vi "Send Message to Azure Queue.vi"() -> ()   [LabVIEW 2015]
doc: "Demonstrates how to send a message to an existing Azure queue."
uses:
  Core/Azure Credentials.ctl
  Core/NI_Azure_Core.lvlib
  Core/Session/Session.lvclass
  Queue/NI_Azure_Queue.lvlib
panel:
  in  "Access Key":string
  in  "Storage Account Name":string
  in  "Queue Name":string
  in  "Message Body":string
  # "Overview: Demonstrates how to send a message to an existing Azure queue.\nRequirements: NI Cloud Toolkit for Azure and a registered Microsoft Azure account\nInstructions:\n1. Specify the Storage Account Name and Access Key for your Azure account. You can create an account at http://azure.microsoft.com.\n2. Specify a Queue Name for the queue to which you want to send a message. You can run the Create New Azure Queue.vi example to create a new queue.\n3. Specify a Message Body to send to the queue.\n4. Run the VI. Verify in the Microsoft Azure Portal that the specified queue has an available message."
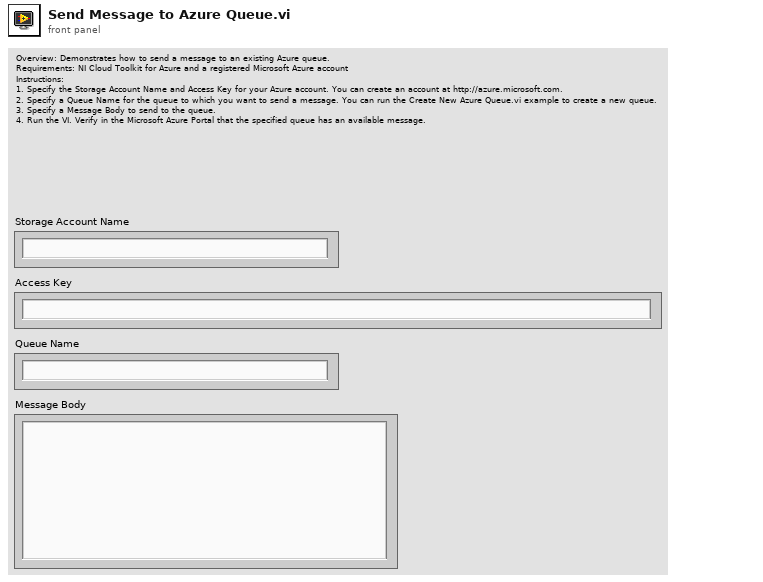
[diagram p1: front panel]
types:
  T1 = typedef "NI_Azure_Core.lvlib/Azure Credentials.ctl" = cluster{"Storage Account Name":string, "Access Key":string}
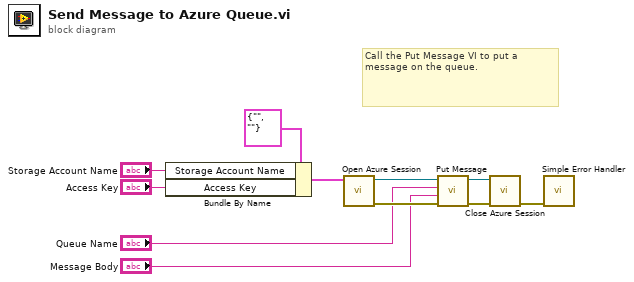
[diagram p0: block diagram]
diagram:
  # "Call the Put Message VI to put a message on the queue."
  n1 = Bundle By Name(cluster=T1 {"Storage Account Name"="", "Access Key"=""} ("Credentials"), "Storage Account Name"="Storage Account Name", "Access Key"="Access Key") -> (w8:T1)
  n2 = call "Open Azure Session.vi"("Credentials"=w8) -> ("error out"=w5:errorcluster, "Azure Session"=w6:refnum<class "Session.lvclass">)  [unwired: 9 in]
  n3 = call "Put Message.vi"("error in (no error)"=w5, "Message"="Message Body", "Queue"="Queue Name", "Azure Session in"=w6) -> ("error out"=w3:errorcluster, "Azure Session out"=w4:refnum<class "Session.lvclass">)  [unwired: 5 in, 1 out]
  n4 = call "Close Azure Session.vi"("error in (no error)"=w3, "Azure Session"=w4) -> ("error out"=w7:errorcluster)  [unwired: 9 in]
  n5 = call <vilib>:"Simple Error Handler.vi"("error in (no error)"=w7) -> ()  [unwired: 4 in, 5 out]
